vi "UI_Elmt_Ref(Label).vi"(8 "error in (no error)":errorcluster, 10 "Elmt Label":string, 11 "UI_Actor in":refnum<class "UI_Actor.lvclass">) -> (0 "error out":errorcluster, 1 "Found":bool, 2 "Ctl Refnum":refnum<vi>, 3 "UI_Actor out":refnum<class "UI_Actor.lvclass">)   [LabVIEW 2020, in "UI_Actor.lvlib" / "UI_Actor.lvclass"]
doc: "Accès à un élément par son label.\n<b> NEVER USE IN FOR LOOP </b> \nLa ref est stockée au premier appel en fgv.\nLe VI doit etre dédié à un unique élement."
uses:
  UI_Actor.lvclass
  UI_Actor.lvclass/UI_Actor.ctl
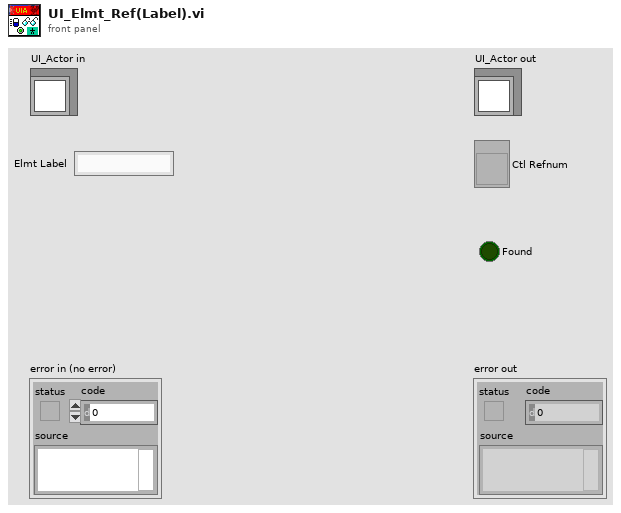
[diagram p1: front panel]
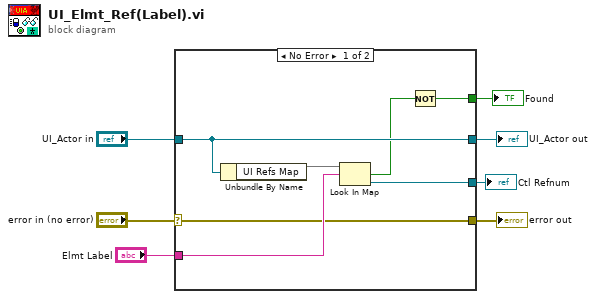
[diagram p0: block diagram]
diagram:
  n1 = case shown="No Error" "error in (no error)" {
    selector: "error in (no error)" -> [w8 w16]
    tunnel: [w8 w16] -> w6
    tunnel: [w14 w15] -> w4
    tunnel: "UI_Actor in" -> [w14 w15]
    tunnel: "Elmt Label" -> [w13 _]
    tunnel: [w11 _] -> w1
    tunnel: [w9 _] -> w2
    frame No Error {
      n2 = Unbundle By Name(w14) -> ("UI Refs Map"=w10:map{string, refnum<vi>})
      n3 = Look In Map(map=w10, key=w13) -> (key not found?=w12:bool, value=w11:refnum<vi>)  [unwired: 1 in]
      n4 = Not(x=w12) -> (.not. x?=w9:bool)
    }
    frame Error {
    }
  }
  "error out" <- w6
  "UI_Actor out" <- w4
  "Found" <- w2
  "Ctl Refnum" <- w1
